vi "setMode.vi"(8 "error in (no error)":errorcluster, 10 "Mode":T1, 11 "Inst.FP in":refnum<class "Inst.FP.lvclass">) -> (0 "error out":errorcluster, 3 "Inst.FP out":refnum<class "Inst.FP.lvclass">)   [LabVIEW 2019, in "Inst.FP.lvclass"]
doc: "Set GHS <b>Mode</b> but pressing a sequence of GHS buttons."
uses:
  Inst.FP.lvclass
  Typedefs/Inst.FP.Modes--Enum.ctl
  Typedefs/Inst.FP.Get Mode--Cluster.ctl
  Typedefs/Inst.FP.Buttons--Enum.ctl
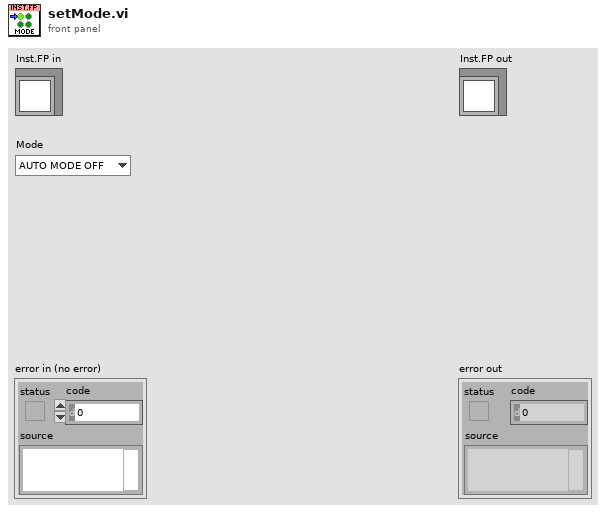
[diagram p1: front panel]
types:
  T1 = typedef "Inst.FP.lvclass/Inst.FP.Modes--Enum.ctl" = enum16{"AUTO MODE OFF", "START", "CONDENSING 3He", "CONDENSING 4He", "NORMAL CIRCULATION", "RECOVERY OF THE MIXTURE", "RECOVERY: BLOCKAGE or OVERPRESSURE"}
  T2 = typedef "Inst.FP.lvclass/Inst.FP.Get Mode--Cluster.ctl" = cluster{"Mode":T1}
  T3 = typedef "Inst.FP.lvclass/Inst.FP.Buttons--Enum.ctl" = enum16{"Start", "3He", "4He", "Normal", "Recovery", "Auto", "LED Test", "Reset"}
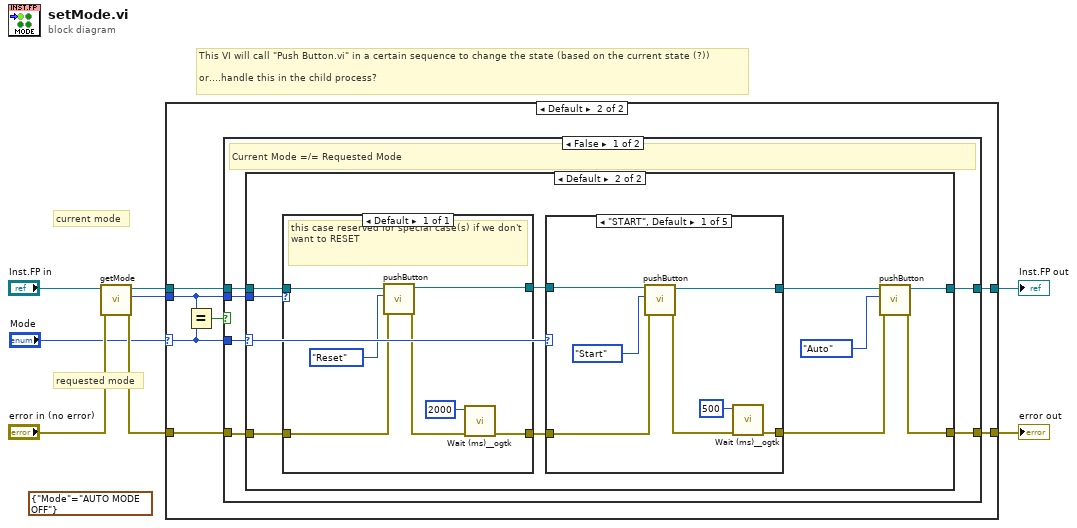
[diagram p0: block diagram]
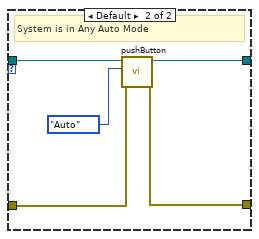
[diagram p4: hidden frame]
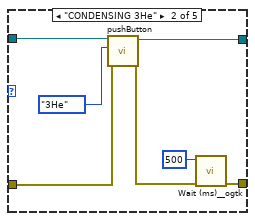
[diagram p5: hidden frame]
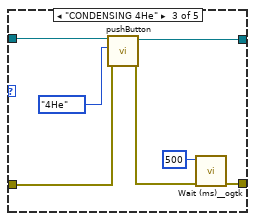
[diagram p6: hidden frame]
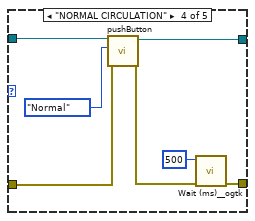
[diagram p7: hidden frame]
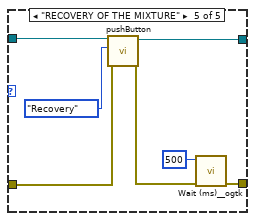
[diagram p8: hidden frame]
diagram:
  (unwired) T2 {"Mode"=enum."AUTO MODE OFF"} ("Get Mode")
  # "requested mode"
  # "current mode"
  # "This VI will call \"Push Button.vi\" in a certain sequence to change the state (based on the current state (?))\n\nor....handle this in the child process?"
  n1 = call-dynamic "getMode.vi"("error in (no error)"="error in (no error)", "Inst.FP in"="Inst.FP in") -> ("error out"=w3:errorcluster, "Mode"=w2:T1, "Inst.FP out"=w5:refnum<class "Inst.FP.lvclass">)  [unwired: 7 in]
  n2 = case shown="Default" "Mode" {
    selector: "Mode" -> [_ w11]
    tunnel: [w9 w17] -> w8
    tunnel: [w10 w16] -> w7
    tunnel: w5 -> [w10 w15]
    tunnel: w3 -> [w9 w14]
    tunnel: w2 -> [_ w13]
    frame "RECOVERY: BLOCKAGE or OVERPRESSURE" {
      # "GHS is in error condition: do not interrupt"
    }
    frame Default {
      n3 = Equal?(x=w13, y=w11) -> (x = y?=w12:bool)
      n4 = case shown="False" w12 {
        tunnel: [w20 w90] -> w17
        tunnel: [w21 w89] -> w16
        tunnel: w15 -> [w23 w89]
        tunnel: w14 -> [w22 w90]
        tunnel: w13 -> [w19 _]
        tunnel: w11 -> [w18 _]
        frame False {
          # "Current Mode =/= Requested Mode"
          n5 = case shown="Default" w18 {
            selector: w18 -> [_ w36]
            tunnel: w23 -> [w28 w46]
            tunnel: w22 -> [w26 w44]
            tunnel: [w27 w42] -> w21
            tunnel: [w25 w39] -> w20
            tunnel: w19 -> [w24 w37]
            frame "AUTO MODE OFF" {
              # "Special Case 1: Turn Off Auto Mode"
              n6 = case shown="\"AUTO MODE OFF\"" w24 {
                tunnel: w28 -> [w30 w34]
                tunnel: [w30 w33] -> w27
                tunnel: w26 -> [w29 w32]
                tunnel: [w29 w31] -> w25
                frame "AUTO MODE OFF" {
                  # "UNLESS Already in Auto Mode Off"
                }
                frame Default {
                  # "System is in Any Auto Mode"
                  n7 = call-dynamic "pushButton.vi"("error in (no error)"=w32, "Button"=Inst.FP.Buttons--Enum."Auto", "Inst.FP"=w34) -> ("error out"=w31:errorcluster, "Inst.FP out"=w33:refnum<class "Inst.FP.lvclass">)  [unwired: 7 in]
                }
              }
            }
            frame Default {
              n8 = case shown="Default" w37 {
                tunnel: w46 -> [w86]
                tunnel: [w85] -> w45
                tunnel: w44 -> [w84]
                tunnel: [w83] -> w40
                frame Default {
                  # "this case reserved for special case(s) if we don't want to RESET"
                  n9 = call-dynamic "pushButton.vi"("error in (no error)"=w84, "Button"=Inst.FP.Buttons--Enum."Reset", "Inst.FP"=w86) -> ("error out"=w82:errorcluster, "Inst.FP out"=w85:refnum<class "Inst.FP.lvclass">)  [unwired: 7 in]
                  n10 = call <userlib>:"Wait (ms)__ogtk.vi"("error in (no error)"=w82, "milliseconds to wait"=u32 2000) -> ("error out"=w83:errorcluster)  [unwired: 8 in, 1 out]
                }
              }
              n11 = case shown="\"START\", Default" w36 {
                tunnel: w45 -> [w50 w57 w64 w71 w78]
                tunnel: [w49 w56 w63 w70 w77] -> w43
                tunnel: [w48 w55 w62 w69 w76] -> w41
                tunnel: w40 -> [w47 w54 w61 w68 w75]
                frame "START", Default {
                  n12 = call-dynamic "pushButton.vi"("error in (no error)"=w47, "Button"=Inst.FP.Buttons--Enum."Start", "Inst.FP"=w50) -> ("error out"=w52:errorcluster, "Inst.FP out"=w49:refnum<class "Inst.FP.lvclass">)  [unwired: 7 in]
                  n13 = call <userlib>:"Wait (ms)__ogtk.vi"("error in (no error)"=w52, "milliseconds to wait"=u32 500) -> ("error out"=w48:errorcluster)  [unwired: 8 in, 1 out]
                }
                frame "CONDENSING 3He" {
                  n14 = call-dynamic "pushButton.vi"("error in (no error)"=w54, "Button"=Inst.FP.Buttons--Enum."3He", "Inst.FP"=w57) -> ("error out"=w59:errorcluster, "Inst.FP out"=w56:refnum<class "Inst.FP.lvclass">)  [unwired: 7 in]
                  n15 = call <userlib>:"Wait (ms)__ogtk.vi"("error in (no error)"=w59, "milliseconds to wait"=u32 500) -> ("error out"=w55:errorcluster)  [unwired: 8 in, 1 out]
                }
                frame "CONDENSING 4He" {
                  n16 = call-dynamic "pushButton.vi"("error in (no error)"=w61, "Button"=Inst.FP.Buttons--Enum."4He", "Inst.FP"=w64) -> ("error out"=w66:errorcluster, "Inst.FP out"=w63:refnum<class "Inst.FP.lvclass">)  [unwired: 7 in]
                  n17 = call <userlib>:"Wait (ms)__ogtk.vi"("error in (no error)"=w66, "milliseconds to wait"=u32 500) -> ("error out"=w62:errorcluster)  [unwired: 8 in, 1 out]
                }
                frame "NORMAL CIRCULATION" {
                  n18 = call-dynamic "pushButton.vi"("error in (no error)"=w68, "Button"=Inst.FP.Buttons--Enum."Normal", "Inst.FP"=w71) -> ("error out"=w73:errorcluster, "Inst.FP out"=w70:refnum<class "Inst.FP.lvclass">)  [unwired: 7 in]
                  n19 = call <userlib>:"Wait (ms)__ogtk.vi"("error in (no error)"=w73, "milliseconds to wait"=u32 500) -> ("error out"=w69:errorcluster)  [unwired: 8 in, 1 out]
                }
                frame "RECOVERY OF THE MIXTURE" {
                  n20 = call-dynamic "pushButton.vi"("error in (no error)"=w75, "Button"=Inst.FP.Buttons--Enum."Recovery", "Inst.FP"=w78) -> ("error out"=w80:errorcluster, "Inst.FP out"=w77:refnum<class "Inst.FP.lvclass">)  [unwired: 7 in]
                  n21 = call <userlib>:"Wait (ms)__ogtk.vi"("error in (no error)"=w80, "milliseconds to wait"=u32 500) -> ("error out"=w76:errorcluster)  [unwired: 8 in, 1 out]
                }
              }
              n22 = call-dynamic "pushButton.vi"("error in (no error)"=w41, "Button"=Inst.FP.Buttons--Enum."Auto", "Inst.FP"=w43) -> ("error out"=w39:errorcluster, "Inst.FP out"=w42:refnum<class "Inst.FP.lvclass">)  [unwired: 7 in]
            }
          }
        }
        frame True {
          # "Current Mode == Requested Mode: Do Nothing"
        }
      }
    }
  }
  "error out" <- w8
  "Inst.FP out" <- w7
